vi "Store Static VI References for Subpanel.vi"(8 "error in (no error)":errorcluster, 11 "Configuration in":refnum<class "GaugeController Configuration.lvclass">) -> (0 "error out":errorcluster, 3 "Configuration out":refnum<class "GaugeController Configuration.lvclass">)   [LabVIEW 2016, in "Hardware.lvlib" / "GaugeController.lvlib" / "GaugeController Configuration.lvclass"]
uses:
  <userlib>/Common Components/Hardware/GaugeController/GaugeController Config/GaugeController Configuration.lvclass
  <userlib>/Configuration Dialog Actor/Configuration.lvclass
  C:/Program Files (x86)/National Instruments/LabVIEW 2016/user.lib/Configuration Dialog Actor/Configuration.lvclass
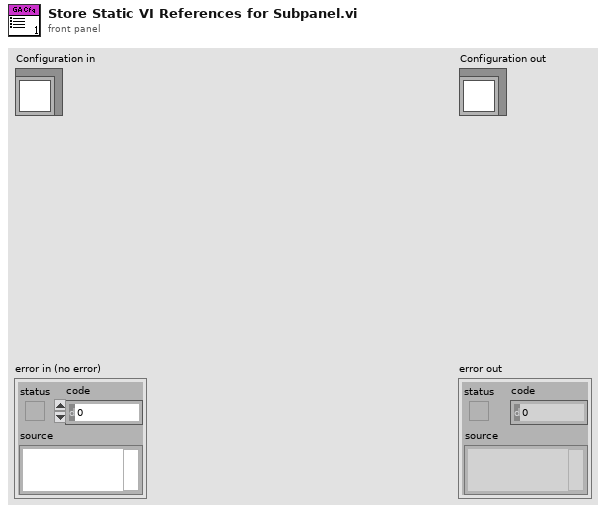
[diagram p1: front panel]
types:
  T1 = typedef "Configuration.lvlib/Configuration.lvclass/Data Retrieved by Lookup Table.ctl" = cluster{"VI Refnum":refnum<vi>, "Help Text":string}
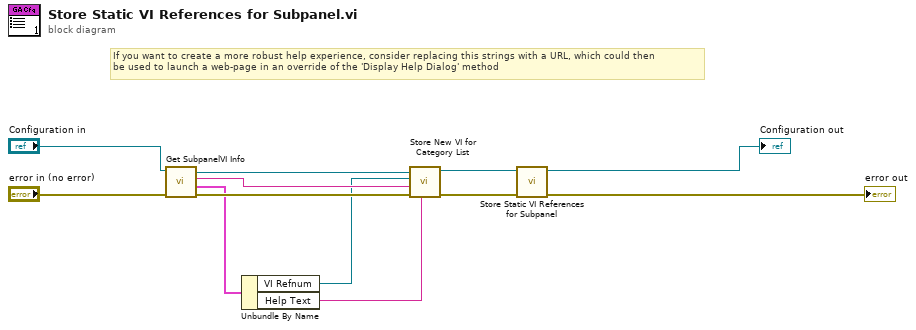
[diagram p0: block diagram]
diagram:
  # "If you want to create a more robust help experience, consider replacing this strings with a URL, which could then\nbe used to launch a web-page in an override of the 'Display Help Dialog' method"
  n1 = call-dynamic "Get SubpanelVI Info.vi"("error in (no error)"="error in (no error)", "GaugeController Configuration in"="Configuration in") -> ("error out"=w5:errorcluster, "Subpanel VI data"=w3:T1, "Category string"=w4:string, "GaugeController Configuration out"=w7:refnum<class "GaugeController Configuration.lvclass">)  [unwired: 6 in]
  n2 = Unbundle By Name(w3) -> ("VI Refnum"=w2:refnum<vi>, "Help Text"=w1:string)
  n3 = call <userlib>:"Store New VI for Category List.vi"("Help Text"=w1, "error in (no error)"=w5, "String"=w4, "VI Refnum"=w2, "Configuration in"=w7) -> ("error out"=w10:errorcluster, "Configuration out"=w11:refnum<class "GaugeController Configuration.lvclass">)  [unwired: 5 in]
  n4 = call-parent "Store Static VI References for Subpanel.vi"("error in (no error)"=w10, "Configuration in"=w11) -> ("error out"=→"error out":errorcluster, "Configuration out"=→"Configuration out":refnum<class "GaugeController Configuration.lvclass">)  [unwired: 8 in]
